vi "VG_TCellmax_P.vi"() -> ()   [LabVIEW 2020]
panel:
  out "TCellmax":dbl
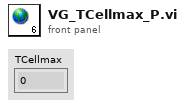
[diagram p1: front panel]
diagram:
